vi "get_consecutive_repetitions.vi"(8 "error in (no error)":errorcluster, 11 "ImagingModeDL090130Frame in":refnum<class "ImagingModeDL090130Frame.lvclass">) -> (0 "error out":errorcluster, 2 "number of consecutive repetitions":i32, 3 "ImagingModeDL090130Frame out":refnum<class "ImagingModeDL090130Frame.lvclass">)   [LabVIEW 2010, in "ImagingModeDL090130Frame.lvclass"]
uses:
  ImagingModeDL090130Frame.lvclass
  ImagingModeDL090130Frame.lvclass/ImagingModeDL090130Frame.ctl
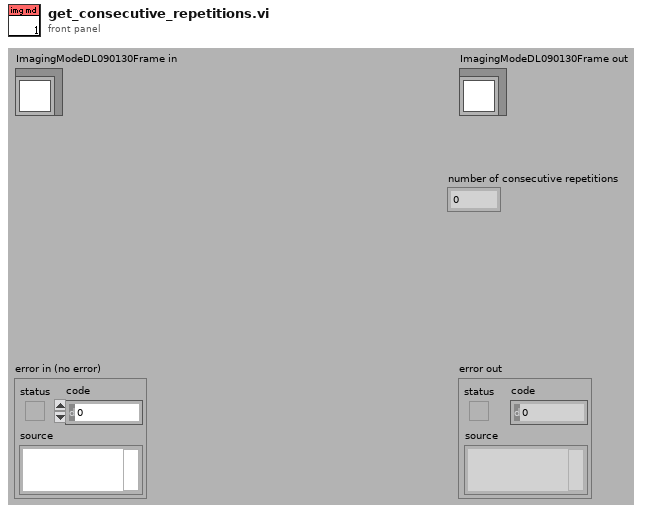
[diagram p1: front panel]
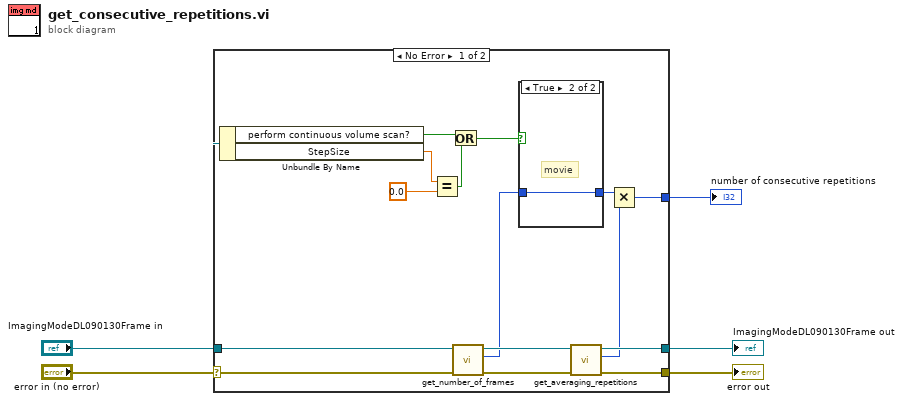
[diagram p0: block diagram]
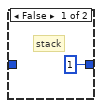
[diagram p2: hidden frame]
diagram:
  n1 = case shown="No Error" "error in (no error)" {
    selector: "error in (no error)" -> [w15 w24]
    tunnel: [w14 w24] -> w4
    tunnel: [w11 w23] -> w3
    tunnel: "ImagingModeDL090130Frame in" -> [w12 w23]
    tunnel: [w6 _] -> w2
    frame No Error {
      n2 = Unbundle By Name(w12) -> ("perform continuous volume scan?"=w17:bool, "StepSize"=w20:dbl[unit])
      n3 = Equal?(x=w20, y=dbl[unit] 0.0 ("settings.StackSettings.StepSize")) -> (x = y?=w18:bool)
      n4 = Or(x=w17, y=w18) -> (x .or. y?=w10:bool)
      n5 = call-dynamic "get_number_of_frames.vi"("error in (no error)"=w15, "ImagingModeDL090130Frame in"=w12) -> ("error out"=w16:errorcluster, "number of frames"=w9:i32, "ImagingModeDL090130Frame out"=w13:refnum<class "ImagingModeDL090130Frame.lvclass">)  [unwired: 7 in]
      n6 = case shown="True" w10 {
        tunnel: w9 -> [_ w22]
        tunnel: [1 ("number of frames") w22] -> w8
        frame False {
          # "stack"
        }
        frame True {
          # "movie"
        }
      }
      n7 = call-dynamic "get_averaging_repetitions.vi"("error in (no error)"=w16, "ImagingModeDL090130Frame in"=w13) -> ("error out"=w14:errorcluster, "averaging repetitions"=w7:i32, "ImagingModeDL090130Frame out"=w11:refnum<class "ImagingModeDL090130Frame.lvclass">)  [unwired: 7 in]
      n8 = Multiply(x=w8, y=w7) -> (x*y=w6:i32)
    }
    frame Error {
    }
  }
  "error out" <- w4
  "ImagingModeDL090130Frame out" <- w3
  "number of consecutive repetitions" <- w2
